vi "Init Arm Pneumatics with CVS File.vi"(10 "Robot ID":string, 11 "Motor ID":string) -> ()   [LabVIEW 2017]
uses:
  <vilib>/Rock Robotics/WPI/SafetyOutput/WPI_SafetyOutputConfigMenu.ctl
  <vilib>/Rock Robotics/WPI/Solenoid/WPI_SolenoidOpenDouble.vi
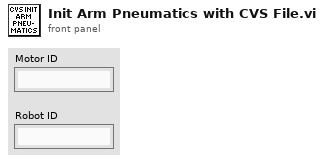
[diagram p1: front panel]
types:
  T1 = typedef "WPI_SafetyOutputConfigMenu.ctl" = enum16{"Enable", "Disable"}
  T2 = typedef "WPI_SolenoidDevRef.ctl" = cluster{"DevStatus":errorcluster, "Pneumatics Control Module":u8, "Forward Solenoid Channel":T3, "Reverse Solenoid Channel":T3}
  T3 = typedef "WPI_SolenoidChannel.ctl" = enum8{"Solenoid 0", "Solenoid 1", "Solenoid 2", "Solenoid 3", "Solenoid 4", "Solenoid 5", "Solenoid 6", "Solenoid 7", "Invalid"}
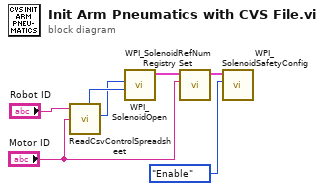
[diagram p0: block diagram]
diagram:
  n1 = call "ReadCsvControlSpreadsheet.vi"("Robot ID"="Robot ID", "Motor ID"="Motor ID") -> ("PDP Channel ID"=w2:i32, "Max Allowed Current"=w3:i32)  [unwired: 1 in, 3 out]
  n2 = call-poly <vilib>:"WPI_SolenoidOpen.vi"("Reverse Solenoid Channel"=w3, "Forward Solenoid Channel"=w2) -> ("SolenoidDevRef"=w4:T2)  [unwired: 8 in, 1 out]
  n3 = call <vilib>:"WPI_SolenoidRefNum Registry Set.vi"("refnum name"="Motor ID", "SolenoidDevRef"=w4) -> ("SolenoidDevRef"=w6:T2)  [unwired: 8 in, 1 out]
  n4 = call <vilib>:"WPI_SolenoidSafetyConfig.vi"("mode"=WPI_SafetyOutputConfigMenu."Enable", "SolenoidDevRef"=w6) -> ()  [unwired: 8 in, 2 out]
